vi "Get Tree Item Position.vi"(10 "Step item":T1, 11 "UI Data in":refnum<class "Settings UI.lvclass">) -> (2 "Position":i32, 3 "UI Data out":refnum<class "Settings UI.lvclass">)   [LabVIEW 2024, in "Output Sequencer.lvlib" / "Settings UI.lvclass"]
uses:
  Settings UI.lvclass
  Types/Tree Index Enum.ctl
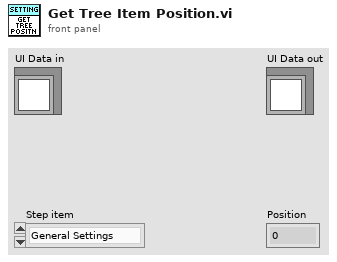
[diagram p1: front panel]
types:
  T1 = typedef "Output Sequencer.lvlib/Settings UI.lvclass/Tree Index Enum.ctl" = enum16{"General Settings", "Num Steps", "Num Analog", "Num Digital", "Show Confirmation", "Interp Priority", "Adv Timing", "Enable Conditions", "Seq Execution", "Reset Test Start", "Only When Test", "Delay After Test", "Start condition", "Re-triggering", "Stop condition", "Stop After Cycles", "Stop Values", "Default Values", "Default Analog", "Default Digital", "Steps", "Step #", "Description", "Precondition", "Duration", "Mode", "Delay Between Vals", "Analog Values", "Digital Values", "Postcondition", "On True", "On False"}
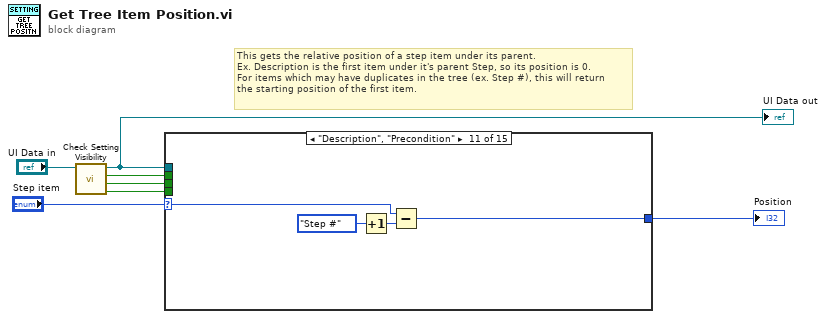
[diagram p0: block diagram]
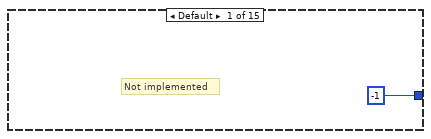
[diagram p2: hidden frame]
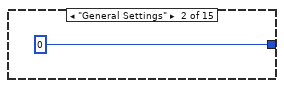
[diagram p3: hidden frame]
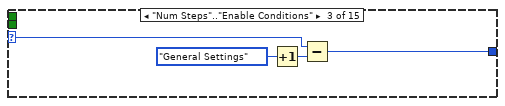
[diagram p4: hidden frame]
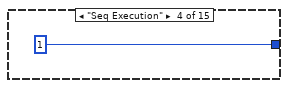
[diagram p5: hidden frame]
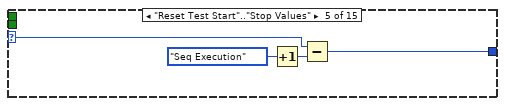
[diagram p6: hidden frame]
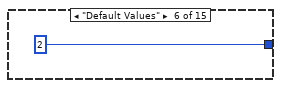
[diagram p7: hidden frame]
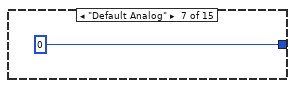
[diagram p8: hidden frame]
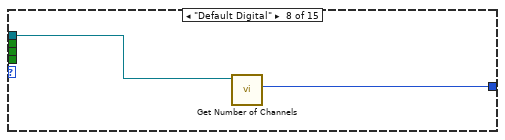
[diagram p9: hidden frame]
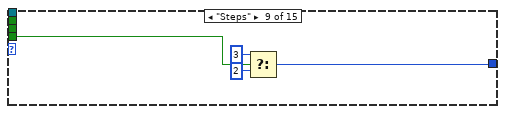
[diagram p10: hidden frame]
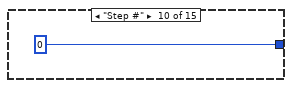
[diagram p11: hidden frame]
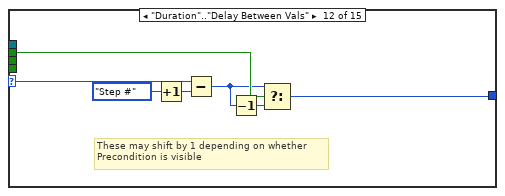
[diagram p12: hidden frame]
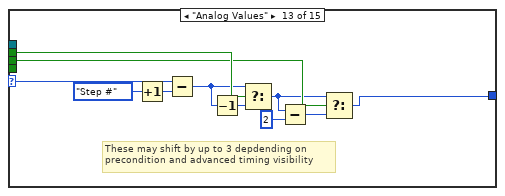
[diagram p13: hidden frame]
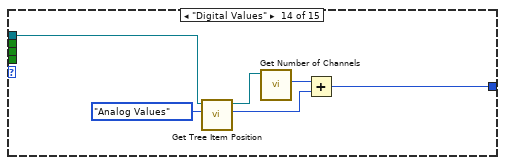
[diagram p14: hidden frame]
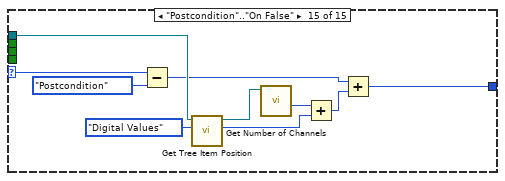
[diagram p15: hidden frame]
diagram:
  # "This gets the relative position of a step item under its parent.\nEx. Description is the first item under it's parent Step, so its position is 0.\nFor items which may have duplicates in the tree (ex. Step #), this will return\nthe starting position of the first item."
  n1 = call "Check Setting Visibility.vi"("UI Data in"="UI Data in") -> ("Channels Visible"=w7:bool, "Advanced timing visible"=w6:bool, "Conditional settings visible"=w5:bool, "UI Data out"=w1:refnum<class "Settings UI.lvclass">)  [unwired: 7 in]
  "UI Data out" <- w1
  n2 = case shown="\"Description\", \"Precondition\"" "Step item" {
    selector: "Step item" -> [_ _ w13 _ w18 _ _ _ _ _ w31 w35 w47 _ w61]
    tunnel: [-1 ("Position") 0 ("Position") w10 1 ("Position") w15 2 ("Position") 0 ("Position") w21 w23 0 ("Position") w28 w36 w39 w50 w56] -> w4
    tunnel: w5 -> [_ _ _ _ _ _ _ _ _ _ _ w37 w48 _ _]
    tunnel: w6 -> [_ _ _ _ _ _ _ _ _ _ _ _ w43 _ _]
    tunnel: w7 -> [_ _ _ _ _ _ _ _ w26 _ _ _ _ _ _]
    tunnel: w1 -> [_ _ _ _ _ _ _ w22 _ _ _ _ _ w55 w65]
    frame Default {
      # "Not implemented"
    }
    frame "General Settings" {
    }
    frame "Num Steps".."Enable Conditions" {
      n3 = Increment(x=Tree_Index_Enum."General Settings" ("y")) -> (x+1=w11:T1)
      n4 = Subtract(x=w13, y=w11) -> (x-y=w10:u16)
    }
    frame "Seq Execution" {
    }
    frame "Reset Test Start".."Stop Values" {
      n5 = Increment(x=Tree_Index_Enum."Seq Execution" ("y")) -> (x+1=w16:T1)
      n6 = Subtract(x=w18, y=w16) -> (x-y=w15:u16)
    }
    frame "Default Values" {
    }
    frame "Default Analog" {
    }
    frame "Default Digital" {
      n7 = call "Get Number of Channels.vi"("UI Data In"=w22) -> ("Num of Analog Channels"=w21:i32)  [unwired: 7 in, 3 out]
    }
    frame "Steps" {
      n8 = Select(t=3 ("Position"), s=w26, f=2 ("Position")) -> (s? t:f=w23:i32)
    }
    frame "Step #" {
    }
    frame "Description", "Precondition" {
      n9 = Increment(x=Tree_Index_Enum."Step #" ("y")) -> (x+1=w29:T1)
      n10 = Subtract(x=w31, y=w29) -> (x-y=w28:u16)
    }
    frame "Duration".."Delay Between Vals" {
      # "These may shift by 1 depending on whether\nPrecondition is visible"
      n11 = Increment(x=Tree_Index_Enum."Step #" ("y")) -> (x+1=w33:T1)
      n12 = Subtract(x=w35, y=w33) -> (x-y=w32:u16)
      n13 = Decrement(x=w32) -> (x-1=w38:u16)
      n14 = Select(t=w32, s=w37, f=w38) -> (s? t:f=w36:u16)
    }
    frame "Analog Values" {
      # "These may shift by up to 3 depdending on\nprecondition and advanced timing visibility"
      n15 = Increment(x=Tree_Index_Enum."Step #" ("y")) -> (x+1=w45:T1)
      n16 = Subtract(x=w47, y=w45) -> (x-y=w44:u16)
      n17 = Decrement(x=w44) -> (x-1=w49:u16)
      n18 = Select(t=w44, s=w48, f=w49) -> (s? t:f=w42:u16)
      n19 = Subtract(x=w42, y=u16 2) -> (x-y=w41:u16)
      n20 = Select(t=w42, s=w43, f=w41) -> (s? t:f=w39:u16)
    }
    frame "Digital Values" {
      n21 = call "Get Tree Item Position.vi"("Step item"=Tree_Index_Enum."Analog Values", "UI Data in"=w55) -> ("Position"=w52:i32, "UI Data out"=w53:refnum<class "Settings UI.lvclass">)  [unwired: 8 in]
      n22 = call "Get Number of Channels.vi"("UI Data In"=w53) -> ("Num of Analog Channels"=w51:i32)  [unwired: 7 in, 3 out]
      n23 = Add(x=w51, y=w52) -> (x+y=w50:i32)
    }
    frame "Postcondition".."On False" {
      n24 = Subtract(x=w61, y=Tree_Index_Enum."Postcondition" ("Step item")) -> (x-y=w58:u16)
      n25 = call "Get Tree Item Position.vi"("Step item"=Tree_Index_Enum."Digital Values", "UI Data in"=w65) -> ("Position"=w62:i32, "UI Data out"=w63:refnum<class "Settings UI.lvclass">)  [unwired: 8 in]
      n26 = call "Get Number of Channels.vi"("UI Data In"=w63) -> ("Num of Digital Channels"=w59:i32)  [unwired: 7 in, 3 out]
      n27 = Add(x=w59, y=w62) -> (x+y=w57:i32)
      n28 = Add(x=w58, y=w57) -> (x+y=w56:i32)
    }
  }
  "Position" <- w4
